vi "Ball Pick Up.vi"(6 "Ball Y":dbl, 7 "Max Speed":dbl, 8 "Ball X":dbl, 9 "Yaw":dbl=1.57, 10 "Speed Setpoint":dbl=0.4, 11 "New Vision Values":bool) -> (1 "Speed Right":dbl, 2 "Speed Left":dbl)   [LabVIEW 2015]
uses:
  Support Code/Team900-VIs/Team900SwerveDrive/Team900SwerveDrive.lvlib
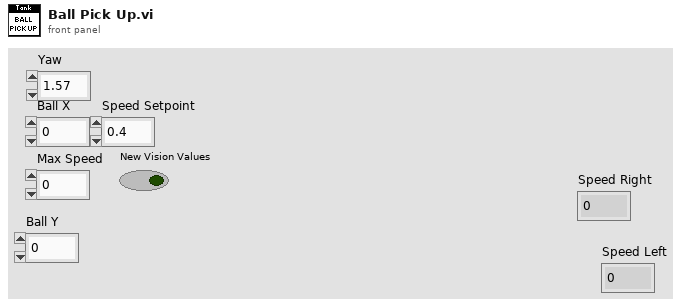
[diagram p1: front panel]
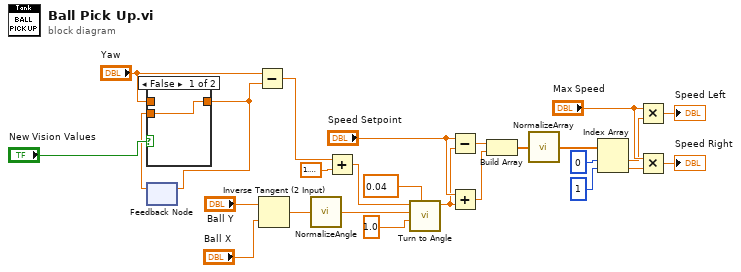
[diagram p0: block diagram]
diagram:
  n1 = feedback #1() -> (w22:dbl)  [unwired: 1 in]
  n2 = case shown="False" "New Vision Values" {
    tunnel: [w27 w28] -> w16
    tunnel: "Yaw" -> [_ w28]
    tunnel: w22 -> [w27 _]
    frame False {
    }
    frame True {
    }
  }
  n3 = feedback-in #1(w16) -> ()
  n4 = Subtract(x="Yaw", y=w16) -> (x-y=w21:dbl)
  n5 = Inverse Tangent (2 Input)(1:"Ball X", 2:"Ball Y") -> (0:w26:dbl)
  n6 = call "NormalizeAngle.vi"("angle (rad)"=w26) -> ("angle (between pi and -pi)"=w11:dbl)
  n7 = Add(x=w21, y=1.5707963267948966) -> (x+y=w19:dbl)
  n8 = call "Turn to Angle.vi"("Angle Tolerance"=0.04, "Rotation Multiplier"=1.0, "Target angle"=w11, "Angle (radians; 0 = right)"=w19) -> ("Turn Set Point"=w12:dbl)  [unwired: 3 in, 1 out]
  n9 = Subtract(x="Speed Setpoint", y=w12) -> (x-y=w10:dbl)
  n10 = Add(x="Speed Setpoint", y=w12) -> (x+y=w3:dbl)
  n11 = Build Array(w10, w3) -> (w9:dbl[])
  n12 = call "NormalizeArray.vi"("array"=w9) -> ("normalized array"=w8:dbl[])
  n13 = Index Array(array=w8, index #1=0 ("index"), index #2=1 ("index")) -> (element #1=w5:dbl, element #2=w4:dbl)
  n14 = Multiply(x="Max Speed", y=w5) -> (x*y=→"Speed Left":dbl)
  n15 = Multiply(x="Max Speed", y=w4) -> (x*y=→"Speed Right":dbl)
